vi "Write TDMS (SubVI).vi"(11 "element":T1) -> (0 "error out":errorcluster, 3 "file path out":path)   [LabVIEW 2017]
uses:
  Vibration.ctl
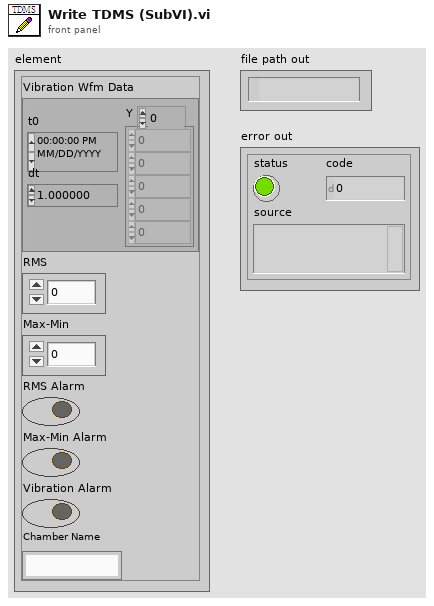
[diagram p1: front panel]
types:
  T1 = typedef "Vibration.ctl" = cluster{"Vibration Wfm Data":waveform(dbl), "RMS":dbl, "Max-Min":dbl, "RMS Alarm":bool, "Max-Min Alarm":bool, "Vibration Alarm":bool, "Chamber Name":string}
  T2 = enum16{"open", "open or create", "create or replace", "create", "open (read-only)"}
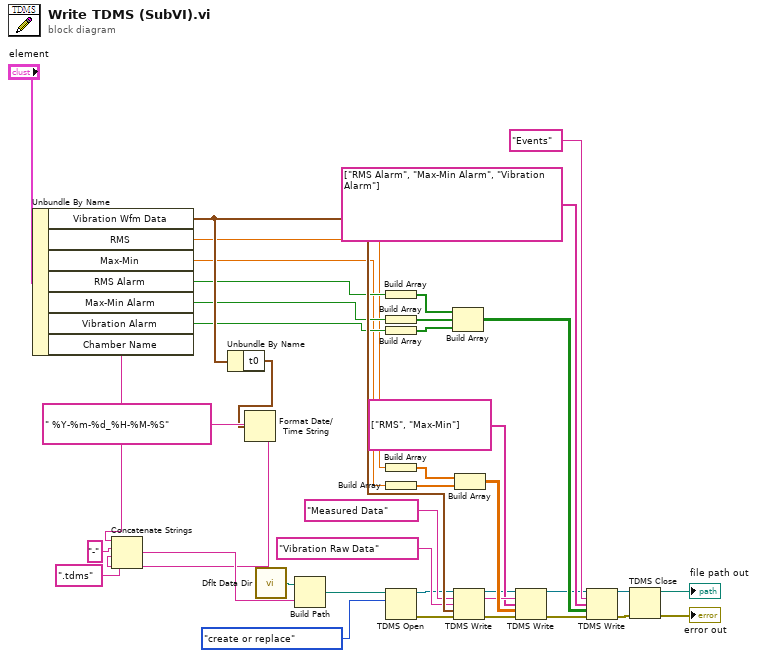
[diagram p0: block diagram]
diagram:
  n1 = Unbundle By Name("element") -> ("Vibration Wfm Data"=w32:waveform(dbl), "RMS"=w16:dbl, "Max-Min"=w17:dbl, "RMS Alarm"=w21:bool, "Max-Min Alarm"=w22:bool, "Vibration Alarm"=w23:bool, "Chamber Name"=w31:string)
  n2 = Unbundle By Name(w32) -> ("t0"=w33:timestamp)
  n3 = Format Date/Time String(time format string (%c)=" %Y-%m-%d_%H-%M-%S", seconds (now)=w33) -> (date/time string=w35:string)  [unwired: 1 in]
  n4 = Concatenate Strings(w31, "-" ("string"), w35, ".tdms" ("string")) -> (w40:string)
  n5 = call <vilib>:"Dflt Data Dir.vi"() -> ("App:Default Data Directory"=w1:path)
  n6 = Build Path(base path=w1, name or relative path=w40) -> (appended path=w2:path)
  n7 = Build Array(w21) -> (w26:bool[])
  n8 = Build Array(w22) -> (w25:bool[])
  n9 = Build Array(w23) -> (w24:bool[])
  n10 = Build Array(w16) -> (w18:dbl[])
  n11 = Build Array(w17) -> (w19:dbl[])
  n12 = TDMS Open(10:T2."create or replace" ("operation (0:open)"), 11:w2) -> (0:w5:errorcluster, 3:w4:refnum<k34>)  [unwired: 5 in]
  n13 = Build Array(w26, w25, w24) -> (w11:bool[][])
  n14 = TDMS Write(0:w4, 5:"Measured Data" ("group name in (Untitled)"), 7:"Vibration Raw Data", 9:w32, 11:w5) -> (4:w9:refnum<k34>, 6:w14:string, 15:w15:errorcluster)  [unwired: 1 in, 1 out]
  n15 = Build Array(w18, w19) -> (w20:dbl[][])
  n16 = TDMS Write(0:w9, 5:w14, 7:string[] ["RMS", "Max-Min"] ("channel name(s) in (Untitled)"), 9:w20, 11:w15) -> (4:w7:refnum<k34>, 15:w8:errorcluster)  [unwired: 1 in, 2 out]
  n17 = TDMS Write(0:w7, 5:"Events" ("group name in (Untitled)"), 7:string[] ["RMS Alarm", "Max-Min Alarm", "Vibration Alarm"] ("channel name(s) in (Untitled)"), 9:w11, 11:w8) -> (4:w12:refnum<k34>, 15:w13:errorcluster)  [unwired: 1 in, 2 out]
  n18 = TDMS Close(8:w13, 11:w12) -> (0:→"error out":errorcluster, 3:→"file path out":path)
